vi "Set CSM State Filter.vi"(10 "CSM:State":cluster{"CSM":string, "State":string}[](array[cluster]), 11 "GlobalLogFilter in":refnum<class "GlobalLogFilter.lvclass">) -> (3 "GlobalLogFilter out":refnum<class "GlobalLogFilter.lvclass">)   [LabVIEW 2017, in "GlobalLogFilter.lvclass"]
uses:
  GlobalLogFilter.lvclass
  GlobalLogFilter.lvclass/GlobalLogFilter.ctl
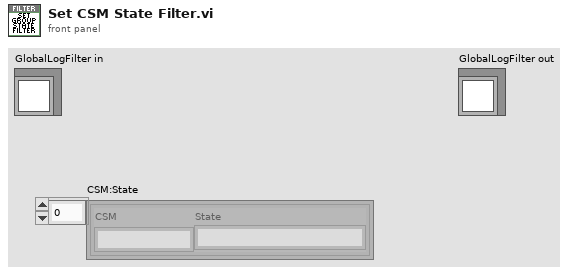
[diagram p1: front panel]
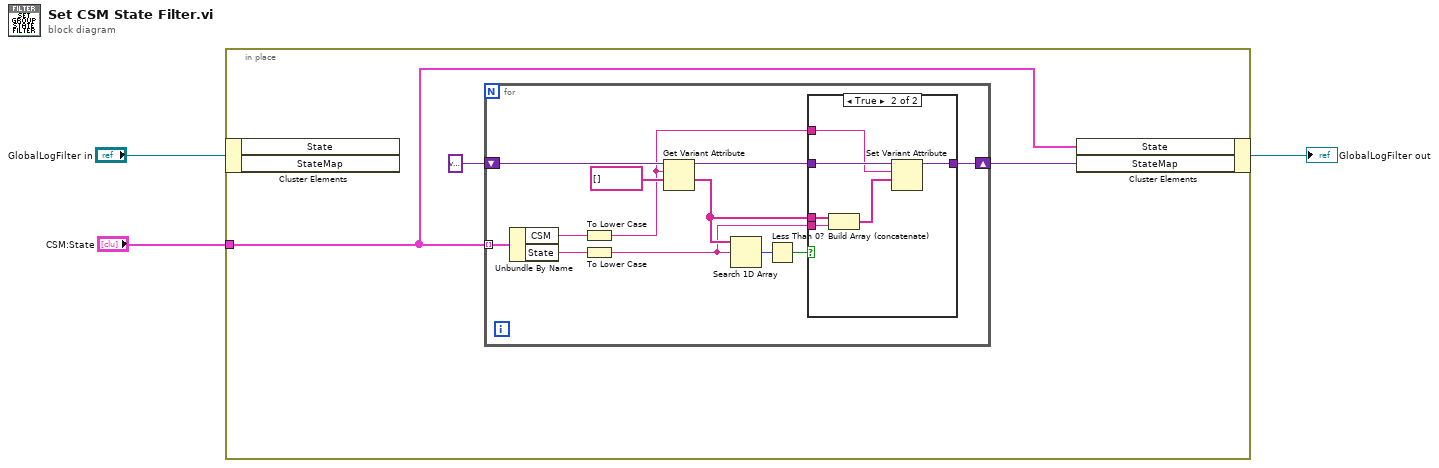
[diagram p0: block diagram]
diagram:
  n1 = in-place "In Place Element Structure" {
    in-place-border: "CSM:State" -> [w4]
    n2 = in-place-cluster #1("GlobalLogFilter in") -> ()  [unwired: 2 out]
    n3 = for {
      shift-right: [w11] -> w5
      shift-left: variant -> [w17]
      tunnel: w4 -> [w18] mode=indexing
      n4 = Unbundle By Name(w18) -> ("CSM"=w10:string, "State"=w12:string)
      n5 = To Lower Case(string=w10) -> (all lower case string=w8:string)
      n6 = To Lower Case(string=w12) -> (all lower case string=w7:string)
      n7 = Get Variant Attribute(Variant=w17, name=w8, default value (empty Variant)=string[] []) -> (duplicate Variant=w16:variant, value=w13:string[])  [unwired: 1 in, 2 out]
      n8 = Search 1D Array(1D array=w13, element=w7) -> (index of element=w14:i32)  [unwired: 1 in]
      n9 = Less Than 0?(x=w14) -> (x < 0?=w9:bool)
      n10 = case shown="True" w9 {
        tunnel: w16 -> [w19 w25]
        tunnel: w13 -> [_ w24]
        tunnel: w7 -> [_ w23]
        tunnel: [w19 w22] -> w11
        tunnel: w8 -> [_ w20]
        frame False {
        }
        frame True {
          n11 = Build Array (concatenate)(w24, w23) -> (w21:string[])
          n12 = Set Variant Attribute(Variant=w25, name=w20, value=w21) -> (Variant out=w22:variant)  [unwired: 1 in, 2 out]
        }
      }
    }
    n13 = in-place-cluster #1("State"=w4, "StateMap"=w5) -> (→"GlobalLogFilter out":refnum<class "GlobalLogFilter.lvclass">)
  }
